vi "Configure Special Pattern Ignore.vi"(8 "error in (no error)":errorcluster, 9 "Ignore Bit Pattern (0: All Bit 0)":i32(ring) items=["All Bit 0", "All Bit 1"], 10 "Enable Special Pattern Ignore (F: Disable)":bool, 11 "VISA resource name":refnum<visa-resource-name>) -> (0 "error out":errorcluster, 3 "VISA resource name out":refnum<visa-resource-name>)   [LabVIEW 2018, in "Agilent PSG MXG Series.lvlib"]
doc: "Configures special pattern ignore function for making BER measurements.\n\n<b>Note:</b>\nIt is applicable for N5172B/82B with <b>Option UN7</b> only."
uses:
  Agilent PSG MXG Series.lvlib
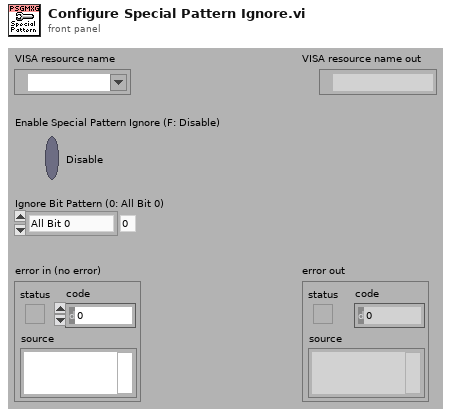
[diagram p1: front panel]
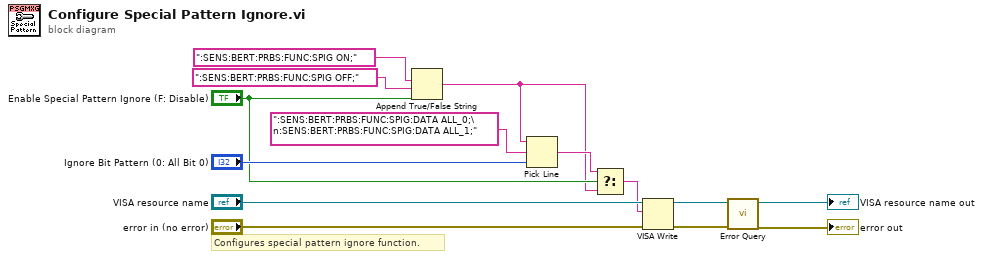
[diagram p0: block diagram]
diagram:
  # "Configures special pattern ignore function."
  n1 = Append True/False String(1:"Enable Special Pattern Ignore (F: Disable)", 2:":SENS:BERT:PRBS:FUNC:SPIG OFF;", 3:":SENS:BERT:PRBS:FUNC:SPIG ON;") -> (0:w1:string)  [unwired: 1 in]
  n2 = Pick Line(string ("")=w1, multi-line string=":SENS:BERT:PRBS:FUNC:SPIG:DATA ALL_0;\n:SENS:BERT:PRBS:FUNC:SPIG:DATA ALL_1;", line index="Ignore Bit Pattern (0: All Bit 0)") -> (output string=w2:string)
  n3 = Select(t=w2, s="Enable Special Pattern Ignore (F: Disable)", f=w1) -> (s? t:f=w4:string)
  n4 = VISA Write(VISA resource name="VISA resource name", write buffer=w4, error in (no error)="error in (no error)") -> (VISA resource name out=w8:refnum<visa-resource-name>, error out=w7:errorcluster)  [unwired: 1 out]
  n5 = call "Error Query.vi"("error in (no error)"=w7, "VISA resource name"=w8) -> ("error out"=→"error out":errorcluster, "VISA resource name out"=→"VISA resource name out":refnum<visa-resource-name>)  [unwired: 6 in, 2 out]
